vi "dfd_Get LV Ver.vi"() -> (0 "LV Version":string)   [LabVIEW 2017, in "NI_DigFilterLicensed.lvlib"]
uses:
  <vilib>/addons/Digital Filter Design/NI_DigFilterLicensed.lvlib
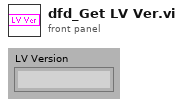
[diagram p1: front panel]
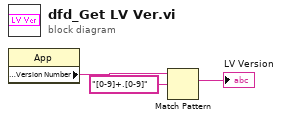
[diagram p0: block diagram]
diagram:
  n1 = property class="App"() -> ("Application:Version Number"=w1:string)  [unwired: 2 in, 2 out]
  n2 = Match Pattern(string=w1, regular expression="[0-9]+.[0-9]") -> (match substring=→"LV Version":string)  [unwired: 1 in, 3 out]
